vi "Begin.vi"(11 "Image Size":T1=enum."160x120") -> (0 "error out":errorcluster)   [LabVIEW 2012]
doc: "Called before other user functions, this VI is expected to open initial I/O refnums, load in file data, and do all program initialization. Notice that the <B>error out</B> terminal is simply used for data flow. Wiring it to other structures or subVIs ensures that this VI runs first."
uses:
  <vilib>/Rock Robotics/WPI/Camera/WPI_CameraImageSize.ctl
  <vilib>/Rock Robotics/SystemInterfaces/DIO/FPGA_DIOPWMChannel.ctl
  <vilib>/Rock Robotics/WPI/Camera/WPI_CameraWhite Balance Values.ctl
  <vilib>/Rock Robotics/WPI/Camera/WPI_CameraExposure Values.ctl
  <vilib>/Rock Robotics/WPI/Camera/WPI_CameraFrameRate.ctl
  <vilib>/Rock Robotics/WPI/DriverStation/WPI_DriverStationRobotMode2.ctl
  <vilib>/Rock Robotics/WPI/Joystick/WPI_JoystickDeviceEnum.ctl
  <vilib>/Rock Robotics/WPI/SafetyOutput/WPI_SafetyOutputConfigMenu.ctl
  <vilib>/Rock Robotics/WPI/RobotDrive/WPI_RobotDriveOpen2MotorWithVictor.vi
  Robot Global Data.vi
  <vilib>/Rock Robotics/WPI/RobotDrive/WPI_RobotDriveOpen2MotorWithTalon.vi
  <vilib>/Rock Robotics/WPI/MotorControl/WPI_MotorControlOpen Talon.vi
  <vilib>/Rock Robotics/WPI/MotorControl/WPI_MotorControlOpen Jaguar.vi
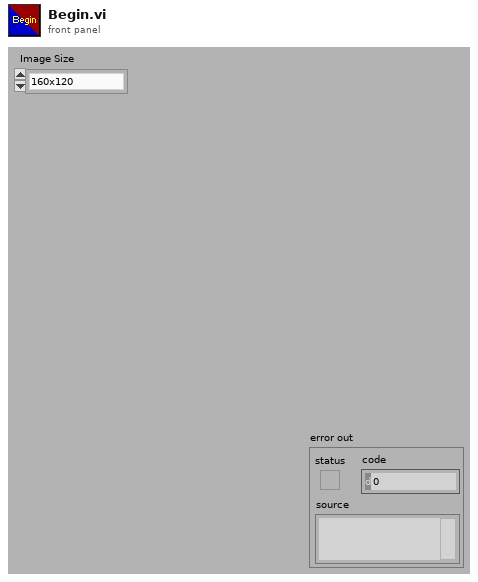
[diagram p1: front panel]
types:
  T1 = typedef "WPI_CameraImageSize.ctl" = enum16{"640x480", "320x240", "160x120"}
  T2 = typedef "WPI_SafetyOutputConfigMenu.ctl" = enum16{"Enable", "Disable"}
  T3 = typedef "FPGA_DIOPWMChannel.ctl" = enum8{"PWM 1", "PWM 2", "PWM 3", "PWM 4", "PWM 5", "PWM 6", "PWM 7", "PWM 8", "PWM 9", "PWM 10", "Invalid"}
  T4 = typedef "WPI_JoystickDeviceEnum.ctl" = enum16{"USB 1", "USB 2", "USB 3", "USB 4", "Kinect 1", "Kinect 2"}
  T5 = typedef "WPI_DriverStationRobotMode2.ctl" = enum16{"Autonomous Disabled", "Autonomous Enabled", "Teleop Disabled", "Teleop Enabled", "Timeout", "Finish", "Test Disabled", "Test Enabled"}
  T6 = typedef "WPI_CameraFrameRate.ctl" = u32
  T7 = typedef "WPI_CameraExposure Values.ctl" = enum16{"Auto", "Flicker-free 50 Hz", "Flicker-free 60 Hz", "Hold current"}
  T8 = typedef "WPI_CameraWhite Balance Values.ctl" = enum16{"Auto", "Fixed indoor", "Fixed outdoor 1", "Fixed outdoor 2", "Fixed fluorescent 1", "Fixed fluorescent 2", "Hold current"}
  T9 = typedef "WPI_CameraDevRef.ctl" = cluster{"Camera Address":string, "CameraStatus":errorcluster, "Acquire Image Notifier":refnum<notifier>}
  T10 = typedef "WPI_JoystickDevRef.ctl" = cluster{"Device":T4}
  T11 = typedef "WPI_RobotDriveDevRef.ctl" = cluster{"DevStatus":errorcluster, "Motors[]":T12[], "Square Inputs":bool, "Max Output":dbl, "Isochronous":bool}
  T12 = typedef "WPI_MotorControlDeviceRef.ctl" = cluster{"DeviceStatus":errorcluster, "Type":enum16{"PWM", "CAN"}, "PWM":cluster{"Digital Module":T13, "PWM Channel":T3, "DeadBand":T14}, "CAN":cluster{"Device Number":u8, "Control Mode":T15, "Semaphore":T16, "Max Vout":dbl}, "Invert":bool, "TransformRef":T17, "InvTransformRef":T17}
  T13 = typedef "FPGA_TypedefDigitalModule.ctl" = enum16{"Digital Module 1", "Digital Module 2"}
  T14 = typedef "WPI_PWMDeadband.ctl" = cluster{"Name":string, "maxPositivePwm":i32, "minPositivePwm":i32, "centerPwm":i32, "maxNegativePwm":i32, "minNegativePwm":i32, "angularRange":u16}
  T15 = typedef "WPI_CANJaguar_ControlMode.ctl" = enum8{"Percent VBus", "Current", "Speed", "Position", "Voltage"}
  T16 = typedef "Semaphore RefNum" = refnum<k1>
  T17 = typedef "WPI_PWMTransform_ConPane.ctl" = refnum<vi>
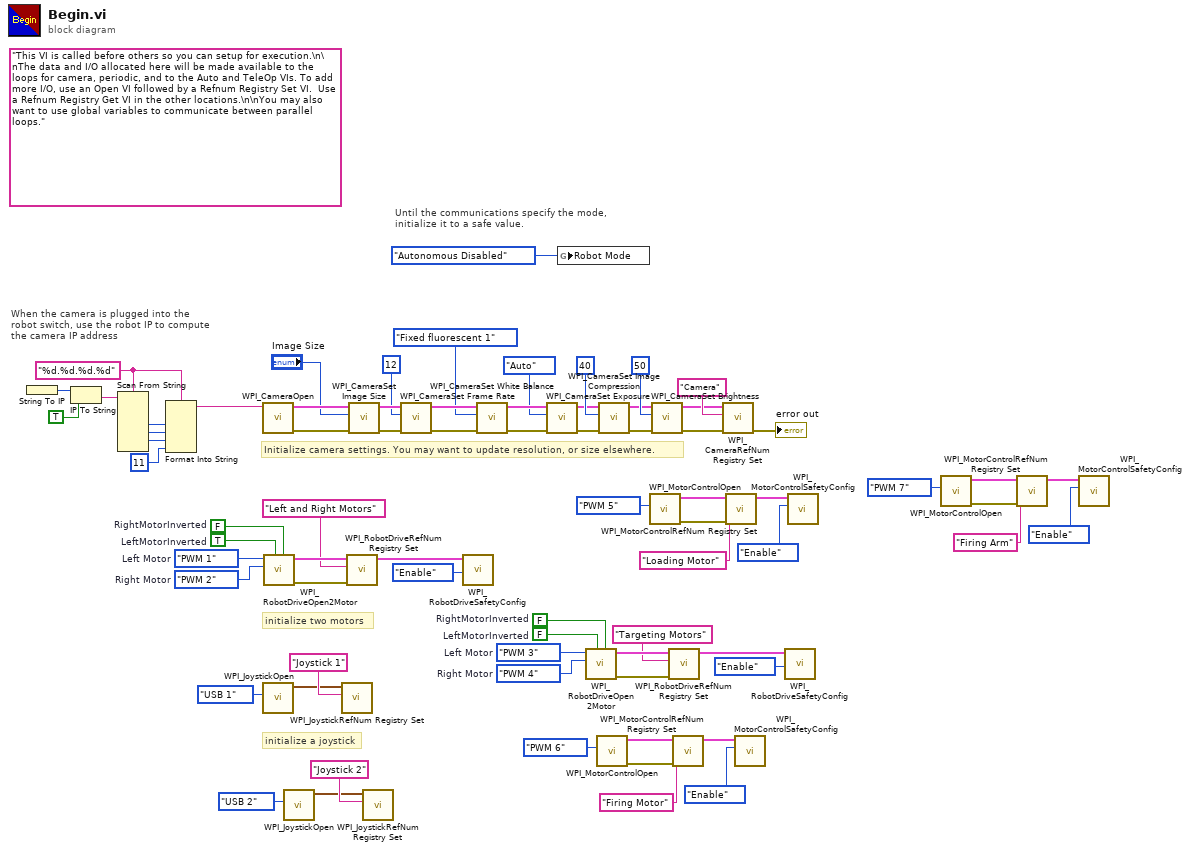
[diagram p0: block diagram]
diagram:
  w24 = FPGA_DIOPWMChannel."PWM 4"  # Right Motor
  w25 = FPGA_DIOPWMChannel."PWM 3"  # Left Motor
  w29 = FALSE  # LeftMotorInverted
  w30 = FALSE  # RightMotorInverted
  w39 = "%d.%d.%d.%d" ("format string")
  (unwired) "This VI is called before others so you can setup for execution.\n\nThe data and I/O allocated here will be made available to the loops for camera, periodic, and to the Auto and TeleOp VIs. To add more I/O, use an Open VI followed by a Refnum Registry Set VI.  Use a Refnum Registry Get VI in the other locations.\n\nYou may also want to use global variables to communicate between parallel loops."
  w50 = FPGA_DIOPWMChannel."PWM 2"  # Right Motor
  w51 = FPGA_DIOPWMChannel."PWM 1"  # Left Motor
  w73 = TRUE  # LeftMotorInverted
  w74 = FALSE  # RightMotorInverted
  # "initialize a joystick"
  # "Until the communications specify the mode,\ninitialize it to a safe value."
  # "When the camera is plugged into the\nrobot switch, use the robot IP to compute\nthe camera IP address"
  # "initialize two motors"
  # "Initialize camera settings. You may want to update resolution, or size elsewhere."
  n1 = String To IP() -> (0:w46:u32)  [unwired: 1 in]
  n2 = IP To String(1:TRUE ("dot notation? (F)"), 2:w46) -> (0:w44:string)
  n3 = Scan From String(format string=w39, input string=w44) -> (output 1=w43:i32, output 2=w42:i32, output 3=w41:i32)  [unwired: 7 in, 3 out]
  n4 = Format Into String(format string=w39, w43, w42, w41, 11 ("Compression")) -> (resulting string=w35:string)  [unwired: 2 in, 1 out]
  n5 = call <vilib>:"WPI_CameraOpen.vi"("Camera Address"=w35) -> ("error out"=w60:errorcluster, "CameraDevRef"=w61:T9)  [unwired: 1 in, 8 out]
  n6 = call <vilib>:"WPI_JoystickOpen.vi"("JoystickDevice"=WPI_JoystickDeviceEnum."USB 1") -> ("JoystickDevRef"=w33:T10)  [unwired: 10 in]
  n7 = call-poly <vilib>:"WPI_RobotDriveOpen2Motor.vi"("Right Motor Inverted"=w74, "Left Motor Inverted"=w73, "Right Motor"=w50, "Left Motor"=w51) -> ("error out"=w69:errorcluster, "RobotDriveDevRef"=w71:T11)  [unwired: 1 in, 5 out]
  n8 = call <vilib>:"WPI_JoystickOpen.vi"("JoystickDevice"=WPI_JoystickDeviceEnum."USB 2") -> ("JoystickDevRef"=w8:T10)  [unwired: 10 in]
  n9 = call <vilib>:"WPI_JoystickRefNum Registry Set.vi"("refnum name"="Joystick 1", "JoystickDevRef"=w33) -> ()  [unwired: 8 in, 2 out]
  n10 = call <vilib>:"WPI_RobotDriveRefNum Registry Set.vi"("error in (no error)"=w69, "refnum name"="Left and Right Motors", "RobotDriveDevRef"=w71) -> ("RobotDriveDevRef"=w38:T11)  [unwired: 8 out]
  n11 = call <vilib>:"WPI_CameraSet Image Size.vi"("error in (no error)"=w60, "Image Size"="Image Size", "CameraDevRef"=w61) -> ("error out"=w59:errorcluster, "CameraDevRef Out"=w62:T9)  [unwired: 7 out]
  n12 = call <vilib>:"WPI_JoystickRefNum Registry Set.vi"("refnum name"="Joystick 2", "JoystickDevRef"=w8) -> ()  [unwired: 8 in, 2 out]
  n13 = call <vilib>:"WPI_CameraSet Frame Rate.vi"("error in (no error)"=w59, "Frame Rate (fps)"=T6 12, "CameraDevRef"=w62) -> ("error out"=w58:errorcluster, "CameraDevRef Out"=w64:T9)  [unwired: 7 out]
  n14 = call <vilib>:"WPI_RobotDriveSafetyConfig.vi"("mode"=WPI_SafetyOutputConfigMenu."Enable", "RobotDriveDevRef"=w38) -> ()  [unwired: 8 in, 2 out]
  n15 = call <vilib>:"WPI_CameraSet White Balance.vi"("error in (no error)"=w58, "White Balance"=WPI_CameraWhite_Balance_Values."Fixed fluorescent 1", "CameraDevRef"=w64) -> ("error out"=w57:errorcluster, "CameraDevRef Out"=w63:T9)  [unwired: 7 out]
  n16 = call <vilib>:"WPI_CameraSet Exposure.vi"("error in (no error)"=w57, "Exposure"=WPI_CameraExposure_Values."Auto", "CameraDevRef"=w63) -> ("error out"=w56:errorcluster, "CameraDevRef Out"=w66:T9)  [unwired: 7 out]
  n17 = global write "Robot Global Data.vi" "Robot Mode"(WPI_DriverStationRobotMode2."Autonomous Disabled" ("Robot Mode")) -> ()
  n18 = call-poly <vilib>:"WPI_RobotDriveOpen2Motor.vi"("Right Motor Inverted"=w30, "Left Motor Inverted"=w29, "Right Motor"=w24, "Left Motor"=w25) -> ("error out"=w26:errorcluster, "RobotDriveDevRef"=w28:T11)  [unwired: 1 in, 5 out]
  n19 = call-poly <vilib>:"WPI_MotorControlOpen.vi"("PWM Channel"=FPGA_DIOPWMChannel."PWM 6") -> ("error out"=w1:errorcluster, "MotorControlDeviceRef"=w5:T12)  [unwired: 9 in]
  n20 = call <vilib>:"WPI_CameraSet Image Compression.vi"("error in (no error)"=w56, "Compression"=40, "CameraDevRef"=w66) -> ("error out"=w55:errorcluster, "CameraDevRef Out"=w65:T9)  [unwired: 7 out]
  n21 = call-poly <vilib>:"WPI_MotorControlOpen.vi"("PWM Channel"=FPGA_DIOPWMChannel."PWM 5") -> ("error out"=w16:errorcluster, "MotorControlDeviceRef"=w20:T12)  [unwired: 9 in]
  n22 = call <vilib>:"WPI_CameraSet Brightness.vi"("error in (no error)"=w55, "Brightness"=50, "CameraDevRef"=w65) -> ("error out"=w53:errorcluster, "CameraDevRef Out"=w54:T9)  [unwired: 7 out]
  n23 = call <vilib>:"WPI_RobotDriveRefNum Registry Set.vi"("error in (no error)"=w26, "refnum name"="Targeting Motors", "RobotDriveDevRef"=w28) -> ("RobotDriveDevRef"=w23:T11)  [unwired: 8 out]
  n24 = call <vilib>:"WPI_MotorControlRefNum Registry Set.vi"("error in (no error)"=w1, "refnum name"="Firing Motor", "MotorControlDevRef"=w5) -> ("MotorControlDevRef"=w3:T12)  [unwired: 7 in, 1 out]
  n25 = call <vilib>:"WPI_CameraRefNum Registry Set.vi"("error in (no error)"=w53, "refnum name"="Camera", "CameraDevRef"=w54) -> ("error out"=→"error out":errorcluster)  [unwired: 8 out]
  n26 = call <vilib>:"WPI_MotorControlRefNum Registry Set.vi"("error in (no error)"=w16, "refnum name"="Loading Motor", "MotorControlDevRef"=w20) -> ("MotorControlDevRef"=w18:T12)  [unwired: 7 in, 1 out]
  n27 = call <vilib>:"WPI_MotorControlSafetyConfig.vi"("mode"=WPI_SafetyOutputConfigMenu."Enable", "MotorControlDevRef"=w3) -> ()  [unwired: 8 in, 2 out]
  n28 = call <vilib>:"WPI_RobotDriveSafetyConfig.vi"("mode"=WPI_SafetyOutputConfigMenu."Enable", "RobotDriveDevRef"=w23) -> ()  [unwired: 8 in, 2 out]
  n29 = call <vilib>:"WPI_MotorControlSafetyConfig.vi"("mode"=WPI_SafetyOutputConfigMenu."Enable", "MotorControlDevRef"=w18) -> ()  [unwired: 8 in, 2 out]
  n30 = call-poly <vilib>:"WPI_MotorControlOpen.vi"("PWM Channel"=FPGA_DIOPWMChannel."PWM 7") -> ("error out"=w10:errorcluster, "MotorControlDeviceRef"=w14:T12)  [unwired: 9 in]
  n31 = call <vilib>:"WPI_MotorControlRefNum Registry Set.vi"("error in (no error)"=w10, "refnum name"="Firing Arm", "MotorControlDevRef"=w14) -> ("MotorControlDevRef"=w12:T12)  [unwired: 7 in, 1 out]
  n32 = call <vilib>:"WPI_MotorControlSafetyConfig.vi"("mode"=WPI_SafetyOutputConfigMenu."Enable", "MotorControlDevRef"=w12) -> ()  [unwired: 8 in, 2 out]
